vi "Simple OpenCreateReplace Dataset (Variant).vi"(4 "Datatype and Dataspace":variant, 5 "Chunk size":i32[](array[numeric]), 6 "operation (open or create)":T1=enum."open or create", 7 "Compression Level (0-disabled)":i32 min=0 max=9 step=1, 8 "error in (no error)":errorcluster, 9 "Unlimited  dataset (F)":bool, 10 "Dataset Path":string, 11 "HDF5 Ref":T2) -> (0 "error out":errorcluster, 2 "HDF5 Dataset Ref out":T2, 3 "HDF5 Ref out":T2)   [LabVIEW 2017]
doc: "Opens, creates or replaces an dataset, using a LabVIEW datatype and specifying additional options."
uses:
  <vilib>/UPVI/lvhdf5/library.llb/HDF5 Ref.ctl
  <vilib>/UPVI/lvhdf5/dataset.llb/LVH5D Operation.ctl
panel:
  # "LVHDF5 Toolkit\nCopyright (c) 2005-2013 by Jason D. Sommerville\nCopyright (c) 2014 by UPVI, LLC.\n\nThis use and distribution of this file is governed by the terms found in \nLICENSE.txt distributed with this toolkit and installed at\n <user.lib>\\_lvhdf5\\LICENSE.txt"
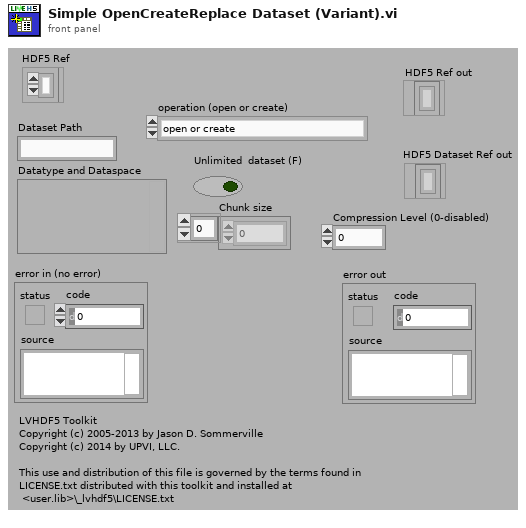
[diagram p1: front panel]
types:
  T1 = typedef "LVH5D Operation.ctl" = enum16{"open", "replace", "create", "open or create", "create or replace", "create or replace with confirmation"}
  T2 = typedef "HDF5 Ref.ctl" = refnum<k1>
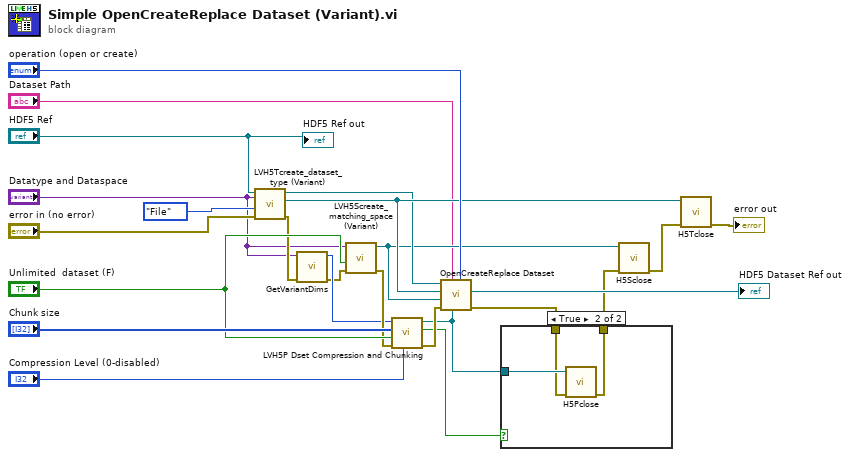
[diagram p0: block diagram]
diagram:
  n1 = call <vilib>:"LVH5Tcreate_dataset_type (Variant).vi"("error in (no error)"="error in (no error)", "Type"=enum16{"File", "Memory"}."File", "Data"="Datatype and Dataspace", "HDF5 Ref"="HDF5 Ref") -> ("error out"=w9:errorcluster, "HDF5 Type Ref"=w20:T2, "HDF5 Ref out"=w18:T2)  [unwired: 3 in, 2 out]
  n2 = call <vilib>:"GetVariantDims.vi"("error in (no error)"=w9, "Variant"="Datatype and Dataspace") -> ("error out"=w7:errorcluster, "rank"=w8:i32)  [unwired: 7 in, 1 out]
  n3 = call <vilib>:"LVH5Screate_matching_space (Variant).vi"("error in (no error)"=w7, "Max size unlimited (F)"="Unlimited  dataset (F)", "Data"="Datatype and Dataspace") -> ("error out"=w11:errorcluster, "HDF5 Dataspace Ref"=w17:T2)  [unwired: 5 in]
  n4 = call <vilib>:"LVH5P Dset Compression and Chunking.vi"("Compression Level (0-disabled)"="Compression Level (0-disabled)", "error in (no error)"=w11, "Unlimited  dataset (F)"="Unlimited  dataset (F)", "Chunk size"="Chunk size", "Dataspace Rank"=w8) -> ("error out"=w14:errorcluster, "Created dcpl?"=w12:bool, "Dataset Creation Property List"=w13:T2)  [unwired: 4 in]
  n5 = call <vilib>:"OpenCreateReplace Dataset.vi"("operation (open or create)"="operation (open or create)", "HDF5 Property List Ref"=w13, "Dataset Path"="Dataset Path", "error in (no error)"=w14, "HDF5 Dataspace Ref"=w17, "HDF5 Datatype Ref"=w20, "HDF5 Ref"=w18) -> ("error out"=w15:errorcluster, "HDF5 Dataset Ref"=→"HDF5 Dataset Ref out":T2)  [unwired: 2 in, 1 out]
  n6 = case shown="True" w12 {
    tunnel: w13 -> [_ w28]
    tunnel: w15 -> [w25 w27]
    tunnel: [w25 w26] -> w16
    frame False {
    }
    frame True {
      n7 = call <vilib>:"H5Pclose.vi"("error in (no error)"=w27, "HDF5 Property Ref"=w28) -> ("error out"=w26:errorcluster)  [unwired: 7 in]
    }
  }
  n8 = call <vilib>:"H5Sclose.vi"("error in (no error)"=w16, "HDF5 Dataspace Ref"=w17) -> ("error out"=w19:errorcluster)  [unwired: 7 in]
  n9 = call <vilib>:"H5Tclose.vi"("error in (no error)"=w19, "HDF5 Datatype Ref"=w20) -> ("error out"=→"error out":errorcluster)  [unwired: 7 in]
  "HDF5 Ref out" <- "HDF5 Ref"
